vi "Initialize Device Core.vi"(8 "error in (no error)":errorcluster, 9 "Reset (F)":bool, 10 "Resource Name":string, 11 "BNT_DAQmx-MCSV in":refnum<class "BNT_DAQmx-MCSV.lvclass">) -> (0 "error out":errorcluster, 3 "BNT_DAQmx-MCSV out":refnum<class "BNT_DAQmx-MCSV.lvclass">)   [LabVIEW 2017, in "BNT_DAQmx.lvlib" / "BNT_DAQmx-MCSV.lvclass"]
doc: "Initialize device driver."
uses:
  BNT_DAQmx-MCSV.lvclass
  C:/User/Brand/LVP/Acc/VacuumHeating/Packages/CSPP_Core/Actors/CSPP_BaseActor/CSPP_BaseActor.lvclass
  CSPP_Core/Actors/CSPP_BaseActor/CSPP_BaseActor.lvclass/CSPP_BaseActor.ctl
  BNT_DAQmx-MCSV.lvclass/BNT_DAQmx-MCSV.ctl
  CSPP_Core/Classes/CSPP_ProcessVariables/PVConnection/PVConnection.lvclass/PVConnection.ctl
  CSPP_Core/Classes/CSPP_ProcessVariables/ProcessVariable/PV.lvclass/PV.ctl
  <vilib>/DAQmx/read.llb/DAQmx Read (Digital 1D Bool 1Chan 1Samp).vi
  CSPP_Core/Classes/CSPP_ProcessVariables/ProcessVariable/Write Data.vi
  CSPP_Core/Classes/CSPP_ProcessVariables/ProcessVariable/Write Error.vi
  CSPP_Core/Classes/CSPP_ProcessVariables/ProcessVariable/Write Quality.vi
  CSPP_Core/Classes/CSPP_ProcessVariables/ProcessVariable/Write status.vi
  CSPP_Core/Classes/CSPP_ProcessVariables/ProcessVariable/Write Timestamp.vi
  <vilib>/DAQmx/read.llb/DAQmx Read (Analog 1D DBL NChan 1Samp).vi
  <vilib>/DAQmx/create/channels.llb/DAQmx Create Channel (DO-Digital Output).vi
  <vilib>/DAQmx/miscellaneous.llb/DAQmx Fill In Error Info.vi
  <vilib>/DAQmx/create/channels.llb/DAQmx Create Channel (DI-Digital Input).vi
  CSPP_Core/Actors/CSPP_DeviceActor/CSPP_DeviceActor.lvclass
  CSPP_Core/Classes/CSPP_ProcessVariables/ProcessVariable/PV.lvclass
  <resource>/objmgr/daqmx.rc
  CSPP_Core/Classes/CSPP_ProcessVariables/PVConnection/PVConnection.lvclass
  CSPP_Core/Actors/CSPP_BaseActor/CSPP_BaseActor.lvclass
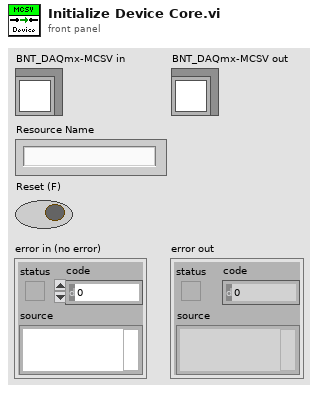
[diagram p1: front panel]
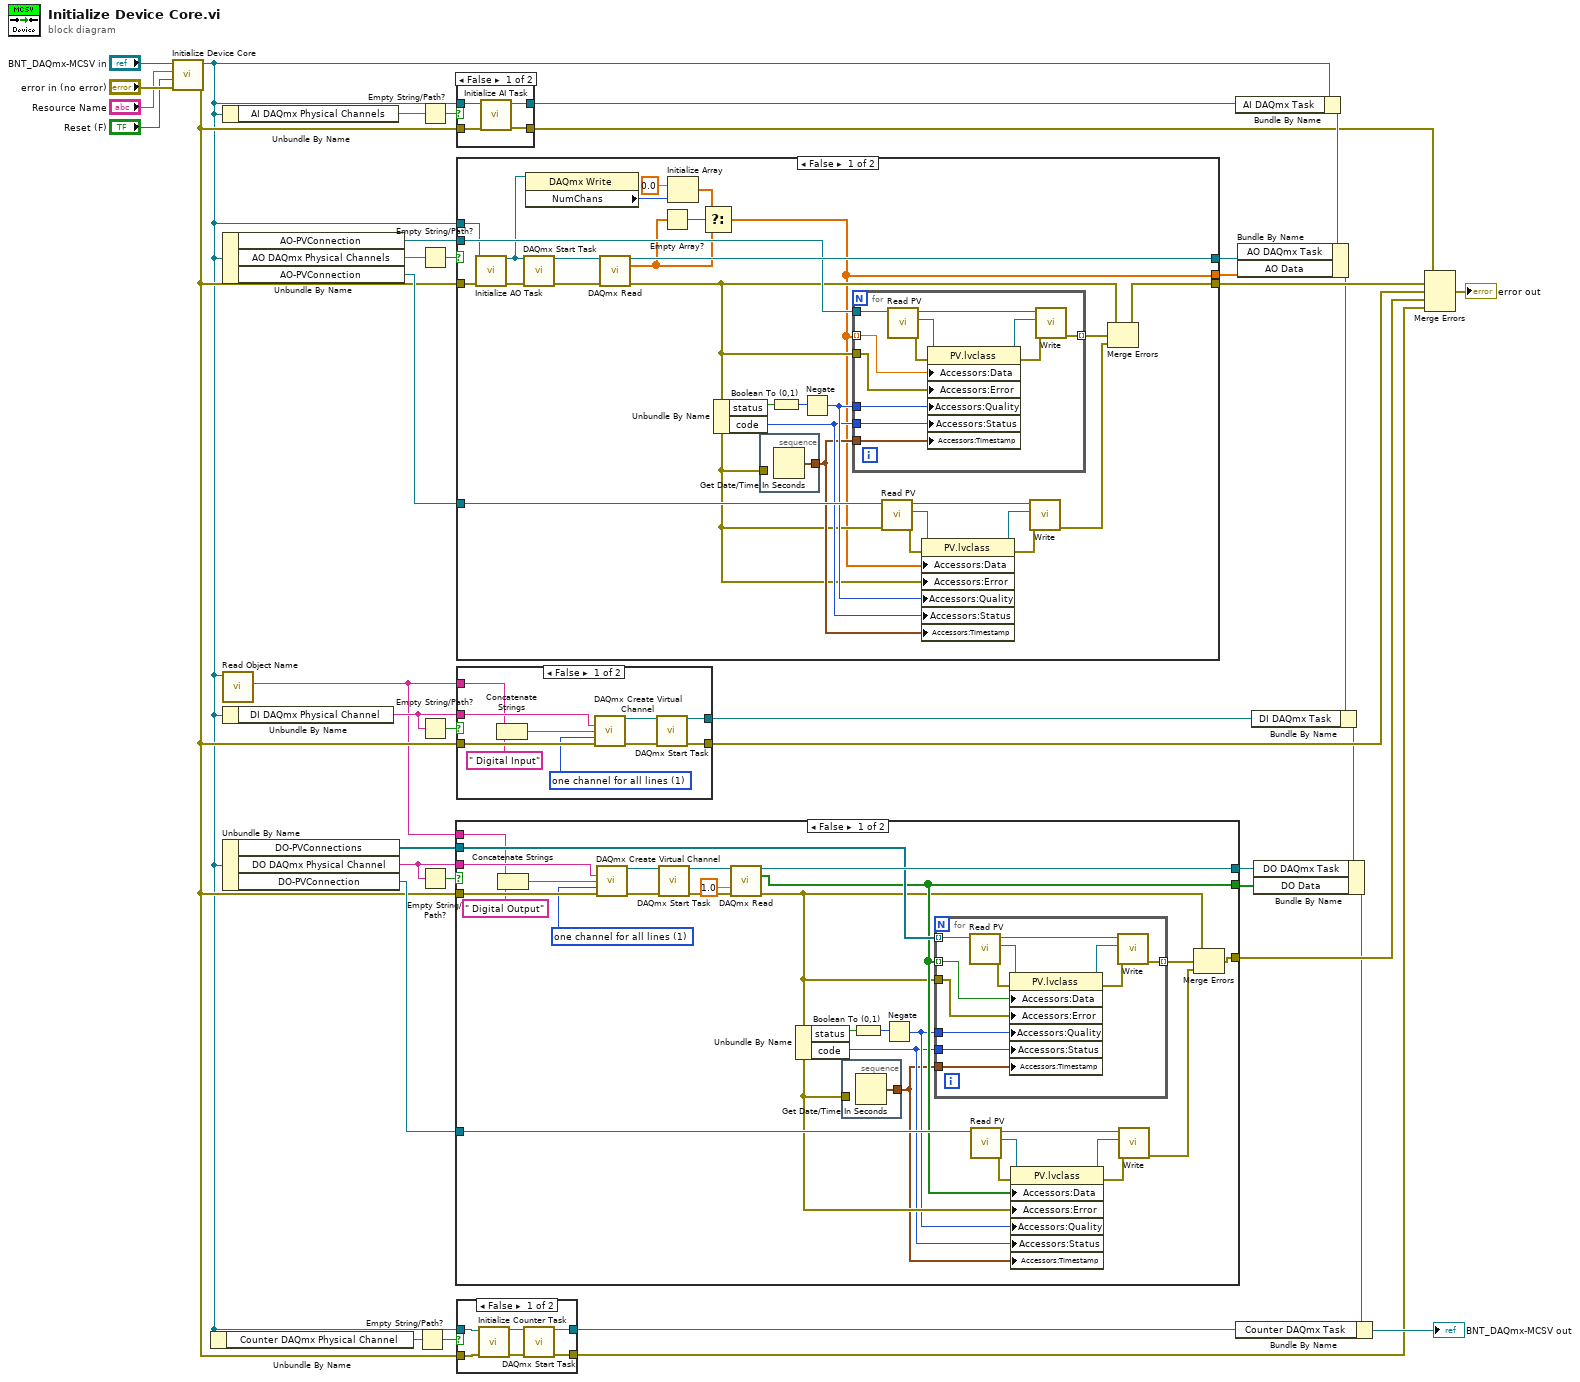
[diagram p0: block diagram]
diagram:
  n1 = call-parent "Initialize Device Core.vi"("error in (no error)"="error in (no error)", "Reset (F)"="Reset (F)", "Resource Name"="Resource Name", "CSPP_DeviceActor in"="BNT_DAQmx-MCSV in") -> ("error out"=w7:errorcluster, "CSPP_DeviceActor out"=w2:refnum<class "BNT_DAQmx-MCSV.lvclass">)  [unwired: 6 in]
  n2 = Unbundle By Name(w2) -> ("Counter DAQmx Physical Channel"=w8:tag)
  n3 = Unbundle By Name(w2) -> ("AI DAQmx Physical Channels"=w29:tag)
  n4 = Unbundle By Name(w2) -> ("AO-PVConnection"=w10:refnum<class "PVConnection.lvclass">, "AO DAQmx Physical Channels"=w27:tag, "AO-PVConnection"=w11:refnum<class "PVConnection.lvclass">)
  n5 = call "Read Object Name.vi"("CSPP_BaseActor in"=w2) -> ("Object Name"=w1:string)  [unwired: 8 in, 2 out]
  n6 = Unbundle By Name(w2) -> ("DI DAQmx Physical Channel"=w24:tag)
  n7 = Unbundle By Name(w2) -> ("DO-PVConnections"=w14:refnum<class "PVConnection.lvclass">[], "DO DAQmx Physical Channel"=w19:tag, "DO-PVConnection"=w12:refnum<class "PVConnection.lvclass">)
  n8 = Empty String/Path?(string/path=w8) -> (empty?=w9:bool)
  n9 = Empty String/Path?(string/path=w29) -> (empty?=w28:bool)
  n10 = Empty String/Path?(string/path=w27) -> (empty?=w26:bool)
  n11 = Empty String/Path?(string/path=w24) -> (empty?=w25:bool)
  n12 = Empty String/Path?(string/path=w19) -> (empty?=w18:bool)
  n13 = case shown="False" w18 {
    tunnel: [w62 _] -> w20
    tunnel: [w55 w82] -> w17
    tunnel: w7 -> [w65 w82]
    tunnel: w19 -> [w63 _]
    tunnel: [w53 _] -> w15
    tunnel: w14 -> [w56 _]
    tunnel: w12 -> [w54 _]
    tunnel: w1 -> [w41 _]
    frame False {
      w64 = 1 items=["one channel for each line", "one channel for all lines"] ("line grouping")
      n14 = Concatenate Strings(w41, " Digital Output" ("string")) -> (w40:string)
      n15 = call-poly <vilib>:"DAQmx Create Virtual Channel.vi"("lines"=w63, "name to assign"=w40, "line grouping"=w64, "error in"=w65) -> ("task out"=w66:refnum<k21>, "error out"=w67:errorcluster)  [unwired: 10 in]
      n16 = call <vilib>:"DAQmx Start Task.vi"("task/channels in"=w66, "error in"=w67) -> ("task out"=w68:refnum<k21>, "error out"=w61:errorcluster)  [unwired: 12 in]
      n17 = call-poly <vilib>:"DAQmx Read.vi"("task/channels in"=w68, "timeout"=1.0, "error in"=w61) -> ("task out"=w62:refnum<k21>, "data"=w53:bool[], "error out"=w52:errorcluster)  [unwired: 10 in]
      n18 = Unbundle By Name(w52) -> ("status"=w58:bool, "code"=w50:i32)
      n19 = stacked-sequence {
        tunnel: [w69] -> w49
        tunnel: w52 -> [_]
        frame #0 {
          n20 = Get Date/Time In Seconds() -> (seconds since 1Jan1904=w69:timestamp)
        }
      }
      n21 = Boolean To (0,1)(Boolean=w58) -> (0, 1=w57:i16)
      n22 = Negate(x=w57) -> (-x=w51:i16)
      n23 = for {
        tunnel: w56 -> [w73] mode=indexing
        tunnel: w53 -> [w81] mode=indexing
        tunnel: w52 -> [w80]
        tunnel: [w77] -> w59 mode=indexing
        tunnel: w51 -> [w76]
        tunnel: w50 -> [w75]
        tunnel: w49 -> [w74]
        n24 = call "Read PV.vi"("PVConnection in"=w73) -> ("error out"=w70:errorcluster, "PV"=w71:refnum<class "PV.lvclass">, "PVConnection out"=w72:refnum<class "PVConnection.lvclass">)  [unwired: 8 in]
        n25 = property class="PV.lvclass"(reference=w71, error in=w70, "Accessors:Data"=w81, "Accessors:Error"=w80, "Accessors:Quality"=w76, "Accessors:Status"=w75, "Accessors:Timestamp"=w74) -> (reference out=w79:refnum<class "PV.lvclass">, error out=w78:errorcluster)
        n26 = call "Write.vi"("error in (no error)"=w78, "PV"=w79, "PVConnection in"=w72) -> ("error out"=w77:errorcluster)  [unwired: 7 in, 1 out]
      }
      n27 = call "Read PV.vi"("PVConnection in"=w54) -> ("error out"=w43:errorcluster, "PV"=w44:refnum<class "PV.lvclass">, "PVConnection out"=w45:refnum<class "PVConnection.lvclass">)  [unwired: 8 in]
      n28 = property class="PV.lvclass"(reference=w44, error in=w43, "Accessors:Data"=w53, "Accessors:Error"=w52, "Accessors:Quality"=w51, "Accessors:Status"=w50, "Accessors:Timestamp"=w49) -> (reference out=w47:refnum<class "PV.lvclass">, error out=w46:errorcluster)
      n29 = call "Write.vi"("error in (no error)"=w46, "PV"=w47, "PVConnection in"=w45) -> ("error out"=w48:errorcluster)  [unwired: 7 in, 1 out]
      n30 = Merge Errors(w52, w59, w48) -> (w55:errorcluster)
    }
    frame True {
    }
  }
  n31 = case shown="False" w28 {
    tunnel: [w84 _] -> w35
    tunnel: w7 -> [w85 w87]
    tunnel: [w83 w87] -> w31
    tunnel: w2 -> [w86 _]
    frame False {
      n32 = call-dynamic "Initialize AI Task.vi"("error in (no error)"=w85, "BNT_DAQmx-MCSV in"=w86) -> ("error out"=w83:errorcluster, "AI DAQmx Task"=w84:refnum<k21>)  [unwired: 8 in]
    }
    frame True {
    }
  }
  n33 = case shown="False" w26 {
    tunnel: [w112 _] -> w34
    tunnel: w7 -> [w97 w129]
    tunnel: [w110 w129] -> w32
    tunnel: [w88 _] -> w13
    tunnel: w10 -> [w111 _]
    tunnel: w11 -> [w104 _]
    tunnel: w2 -> [w96 _]
    frame False {
      n34 = call-dynamic "Initialize AO Task.vi"("error in (no error)"=w97, "BNT_DAQmx-MCSV in"=w96) -> ("error out"=w98:errorcluster, "AO DAQmx Task"=w94:refnum<k21>)  [unwired: 8 in]
      n35 = call <vilib>:"DAQmx Start Task.vi"("task/channels in"=w94, "error in"=w98) -> ("task out"=w95:refnum<k21>, "error out"=w99:errorcluster)  [unwired: 12 in]
      n36 = property class="DAQmx Write"(reference=w94) -> ("NumChans"=w93:u32)  [unwired: 1 in, 2 out]
      n37 = call-poly <vilib>:"DAQmx Read.vi"("task/channels in"=w95) -> ("task out"=w112:refnum<k21>, "data"=w89:dbl[])  [unwired: 12 in, 1 out]
      n38 = Empty Array?(array=w89) -> (empty?=w91:bool)
      n39 = Initialize Array(0.0 ("element"), w93) -> (w90:dbl[])
      n40 = Select(t=w90, s=w91, f=w89) -> (s? t:f=w88:dbl[])
      n41 = Unbundle By Name(w99) -> ("status"=w114:bool, "code"=w102:i32)
      n42 = stacked-sequence {
        tunnel: [w116] -> w101
        tunnel: w99 -> [_]
        frame #0 {
          n43 = Get Date/Time In Seconds() -> (seconds since 1Jan1904=w116:timestamp)
        }
      }
      n44 = Boolean To (0,1)(Boolean=w114) -> (0, 1=w115:i16)
      n45 = Negate(x=w115) -> (-x=w103:i16)
      n46 = for {
        tunnel: w111 -> [w120]
        tunnel: w88 -> [w128] mode=indexing
        tunnel: w99 -> [w127]
        tunnel: [w124] -> w113 mode=indexing
        tunnel: w103 -> [w123]
        tunnel: w102 -> [w122]
        tunnel: w101 -> [w121]
        n47 = call "Read PV.vi"("PVConnection in"=w120) -> ("error out"=w117:errorcluster, "PV"=w118:refnum<class "PV.lvclass">, "PVConnection out"=w119:refnum<class "PVConnection.lvclass">)  [unwired: 8 in]
        n48 = property class="PV.lvclass"(reference=w118, error in=w117, "Accessors:Data"=w128, "Accessors:Error"=w127, "Accessors:Quality"=w123, "Accessors:Status"=w122, "Accessors:Timestamp"=w121) -> (reference out=w126:refnum<class "PV.lvclass">, error out=w125:errorcluster)
        n49 = call "Write.vi"("error in (no error)"=w125, "PV"=w126, "PVConnection in"=w119) -> ("error out"=w124:errorcluster)  [unwired: 7 in, 1 out]
      }
      n50 = call "Read PV.vi"("error in (no error)"=w99, "PVConnection in"=w104) -> ("error out"=w109:errorcluster, "PV"=w108:refnum<class "PV.lvclass">, "PVConnection out"=w107:refnum<class "PVConnection.lvclass">)  [unwired: 7 in]
      n51 = property class="PV.lvclass"(reference=w108, error in=w109, "Accessors:Data"=w88, "Accessors:Error"=w99, "Accessors:Quality"=w103, "Accessors:Status"=w102, "Accessors:Timestamp"=w101) -> (reference out=w105:refnum<class "PV.lvclass">, error out=w106:errorcluster)
      n52 = call "Write.vi"("error in (no error)"=w106, "PV"=w105, "PVConnection in"=w107) -> ("error out"=w100:errorcluster)  [unwired: 7 in, 1 out]
      n53 = Merge Errors(w99, w113, w100) -> (w110:errorcluster)
    }
    frame True {
    }
  }
  n54 = case shown="False" w25 {
    tunnel: [w139 _] -> w22
    tunnel: [w136 w140] -> w21
    tunnel: w7 -> [w135 w140]
    tunnel: w24 -> [w133 _]
    tunnel: w1 -> [w132 _]
    frame False {
      w134 = 1 items=["one channel for each line", "one channel for all lines"] ("line grouping")
      n55 = Concatenate Strings(w132, " Digital Input" ("string")) -> (w131:string)
      n56 = call-poly <vilib>:"DAQmx Create Virtual Channel.vi"("lines"=w133, "name to assign"=w131, "line grouping"=w134, "error in"=w135) -> ("task out"=w137:refnum<k21>, "error out"=w138:errorcluster)  [unwired: 10 in]
      n57 = call <vilib>:"DAQmx Start Task.vi"("task/channels in"=w137, "error in"=w138) -> ("task out"=w139:refnum<k21>, "error out"=w136:errorcluster)  [unwired: 12 in]
    }
    frame True {
    }
  }
  n58 = case shown="False" w9 {
    tunnel: [w146 _] -> w5
    tunnel: w7 -> [w143 w147]
    tunnel: [w145 w147] -> w3
    tunnel: w2 -> [w144 _]
    frame False {
      n59 = call-dynamic "Initialize Counter Task.vi"("error in (no error)"=w143, "BNT_DAQmx-MCSV in"=w144) -> ("error out"=w141:errorcluster, "Counter DAQmx Task"=w142:refnum<k21>)  [unwired: 8 in]
      n60 = call <vilib>:"DAQmx Start Task.vi"("task/channels in"=w142, "error in"=w141) -> ("task out"=w146:refnum<k21>, "error out"=w145:errorcluster)  [unwired: 12 in]
    }
    frame True {
    }
  }
  n61 = Bundle By Name(cluster=w2, "AI DAQmx Task"=w35) -> (w33:refnum<class "BNT_DAQmx-MCSV.lvclass">)
  n62 = Bundle By Name(cluster=w33, "AO DAQmx Task"=w34, "AO Data"=w13) -> (w23:refnum<class "BNT_DAQmx-MCSV.lvclass">)
  n63 = Bundle By Name(cluster=w23, "DI DAQmx Task"=w22) -> (w16:refnum<class "BNT_DAQmx-MCSV.lvclass">)
  n64 = Bundle By Name(cluster=w16, "DO DAQmx Task"=w20, "DO Data"=w15) -> (w6:refnum<class "BNT_DAQmx-MCSV.lvclass">)
  n65 = Bundle By Name(cluster=w6, "Counter DAQmx Task"=w5) -> (→"BNT_DAQmx-MCSV out":refnum<class "BNT_DAQmx-MCSV.lvclass">)
  n66 = Merge Errors(w31, w32, w21, w17, w3) -> (→"error out":errorcluster)
